vi "appendNewRecordString.vi"(0 "New Record String":string, 1 "clear":bool, 2 "Level":T1(ring), 3 "Style Color":u32[](array[colorbox])) -> (4 "Log Display Updated":string, 6 "Colors":cluster{"length":u32, "color":u32}[](array[cluster]))   [LabVIEW 2017, in "Error Log.lvlib" / "Handler.UserEvent.Console.lvclass"]
uses:
  Handler.UserEvent.Console.lvclass
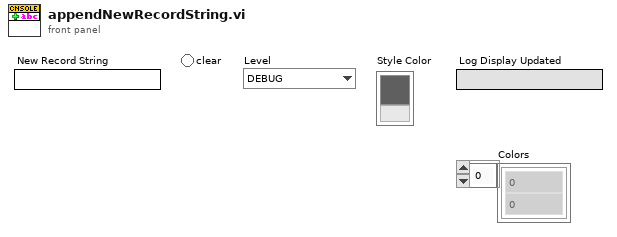
[diagram p1: front panel]
types:
  T1 = enum16{"DEBUG", "INFO", "WARNING", "ERROR", "CRITICAL"}
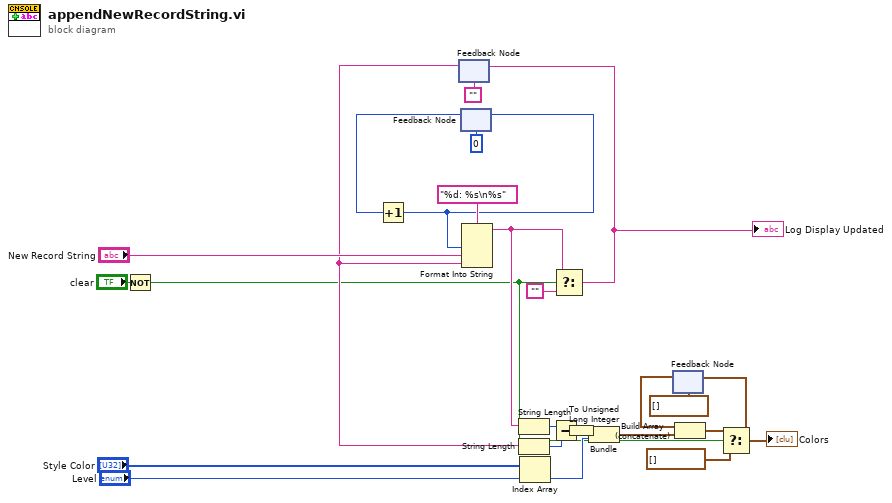
[diagram p0: block diagram]
diagram:
  n1 = Not(x="clear") -> (.not. x?=w5:bool)
  n2 = feedback #1("") -> (w12:string)
  n3 = feedback #2(0) -> (w23:i32)
  n4 = Increment(x=w23) -> (x+1=w22:i32)
  n5 = feedback-in #2(w22) -> ()
  n6 = Format Into String(format string="%d: %s\n%s", w22, "New Record String", w12) -> (resulting string=w13:string)  [unwired: 2 in, 1 out]
  n7 = String Length(string=w13) -> (length=w16:i32)
  n8 = String Length(string=w12) -> (length=w11:i32)
  n9 = Index Array(array="Style Color", index="Level") -> (element=w6:u32)
  n10 = Subtract(x=w16, y=w11) -> (x-y=w10:i32)
  n11 = Select(t=w13, s=w5, f="") -> (s? t:f=w18:string)
  "Log Display Updated" <- w18
  n12 = feedback-in #1(w18) -> ()
  n13 = To Unsigned Long Integer(number=w10) -> (unsigned 32bit integer=w9:u32)
  n14 = Bundle(w9, "Color Box"=w6) -> (w15:cluster{u32, "Color Box":u32})  [unwired: 1 in]
  n15 = feedback #3(cluster{"length":u32, "Color":u32}[] []) -> (w14:cluster{"length":u32, "Color":u32}[])
  n16 = Build Array (concatenate)(w14, w15) -> (w4:cluster{"length":u32, "Color Box":u32}[])
  n17 = Select(t=w4, s=w5, f=cluster{"length":u32, "Color Box":u32}[] []) -> (s? t:f=w3:cluster{"length":u32, "Color Box":u32}[])
  "Colors" <- w3
  n18 = feedback-in #3(w3) -> ()
